vi "process.vi"(8 "error in":errorcluster, 9 "result allocation":T1, 10 "parameters":T1, 11 "module in":refnum<class "PID Module runtime.lvclass">) -> (0 "error out":errorcluster, 1 "results":T1, 2 "parameter allocation":T1, 3 "module out":refnum<class "PID Module runtime.lvclass">)   [LabVIEW 2015, in "PID Module runtime.lvclass"]
doc: "Provides an interface for information processing by a module at runtime. While this interface performs no operations, a child should provide an override which may process data in any manner necessary."
uses:
  PID Module runtime.lvclass
  <vilib>/NI/Tag Bus/table/data table.ctl
  PID Module runtime.lvclass/PID Module runtime.ctl
  <vilib>/NI/Tag Bus/table/data polymorphs/write many/write Doubles.vi
  <vilib>/addons/control/pid/pid.llb/PID (DBL Array).vi
  <vilib>/addons/control/pid/NI_PID_pid.lvlib
  <vilib>/NI/Tag Bus/table/data table.lvlib
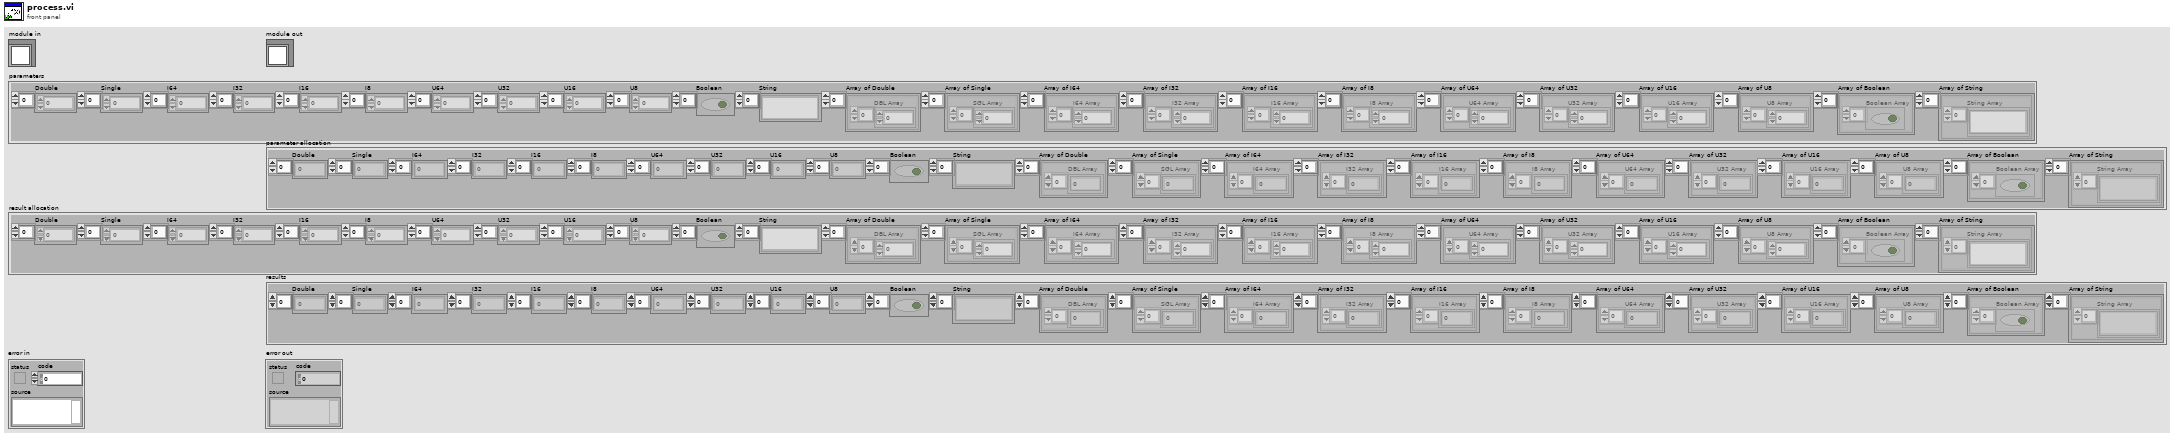
[diagram p1: front panel]
types:
  T1 = typedef "tag bus.lvlib/data table.lvlib/data table.ctl" = cluster{"Double":dbl[], "Single":sgl[], "I64":i64[], "I32":i32[], "I16":i16[], "I8":i8[], "U64":u64[], "U32":u32[], "U16":u16[], "U8":u8[], "Boolean":bool[], "String":string[], "Array of Double":cluster{"DBL Array":dbl[]}[], "Array of Single":cluster{"SGL Array":sgl[]}[], "Array of I64":cluster{"I64 Array":i64[]}[], "Array of I32":cluster{"I32 Array":i32[]}[], "Array of I16":cluster{"I16 Array":i16[]}[], "Array of I8":cluster{"I8 Array":i8[]}[], "Array of U64":cluster{"U64 Array":u64[]}[], "Array of U32":cluster{"U32 Array":u32[]}[], "Array of U16":cluster{"U16 Array":u16[]}[], "Array of U8":cluster{"U8 Array":u8[]}[], "Array of Boolean":cluster{"Boolean Array":bool[]}[], "Array of String":cluster{"String Array":string[]}[]}
  T2 = typedef "PID Module runtime.lvclass/Mapping.ctl" = cluster{"Setpoints":i32[], "Variable":i32[], "Output":i32[], "High":i32[], "Low":i32[], "P":i32[], "I":i32[], "D":i32[]}
  T3 = typedef "PID Module runtime.lvclass/PID Parameters.ctl" = cluster{"Setpoints":dbl[], "Process Variables":dbl[], "output range":cluster{"output high":dbl, "output low":dbl}[], "PID gains":cluster{"proportional gain (Kc)":dbl, "integral time (Ti, min)":dbl, "derivative time (Td, min)":dbl}[]}
  T4 = cluster{"proportional gain (Kc)":dbl, "integral time (Ti, min)":dbl, "derivative time (Td, min)":dbl}[]
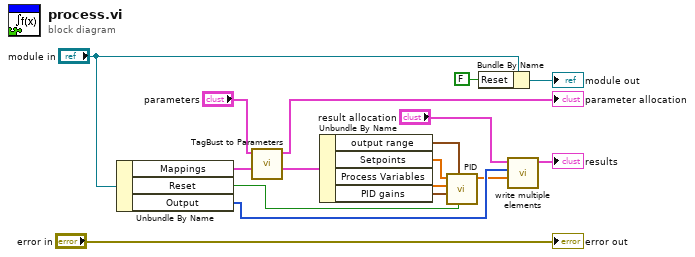
[diagram p0: block diagram]
diagram:
  n1 = Unbundle By Name("module in") -> ("Mappings"=w11:T2, "Reset"=w16:bool, "Output"=w5:i32[])
  n2 = call "TagBust to Parameters.vi"("Mapping"=w11, "parameters"="parameters") -> ("PID Parameters"=w10:T3, "data table out"=→"parameter allocation":T1)  [unwired: 8 in]
  n3 = Unbundle By Name(w10) -> ("output range"=w6:cluster{"output high":dbl, "output low":dbl}[], "Setpoints"=w9:dbl[], "Process Variables"=w8:dbl[], "PID gains"=w7:T4)
  n4 = call-poly <vilib>:"PID.vi"("reinitialize? (F)"=w16, "output range"=w6, "PID gains"=w7, "process variable"=w8, "setpoint"=w9) -> ("output"=w4:dbl[])  [unwired: 5 in, 1 out]
  n5 = Bundle By Name(cluster="module in", "Reset"=FALSE) -> (→"module out":refnum<class "PID Module runtime.lvclass">)
  n6 = call-poly <vilib>:"write multiple elements.vi"("values"=w4, "indices"=w5, "data table in"="result allocation") -> ("data table out"=→"results":T1)  [unwired: 8 in]
  "error out" <- "error in"
